vi "build status string.vi"(1 "SpyMessage{}":T1 {"AckBytes [8]" format="%.0x"; "Data [8]" format="%.0x"; "ArbIDOrHeader" format="%.0x"; "DescriptionID" format="%.0x"; "NetworkID" format="%.0x"}, 2 "timestamp":dbl) -> (0 "string out":string)   [LabVIEW 2009]
doc: "this vi builds the string that to be displayed from the received messages.\n\n1/04/2010 1.0.0 jyg\n-initial release"
uses:
  ctl spymessage.ctl
  ctl StatusBitfield.ctl
  ctl spy protocols.ctl
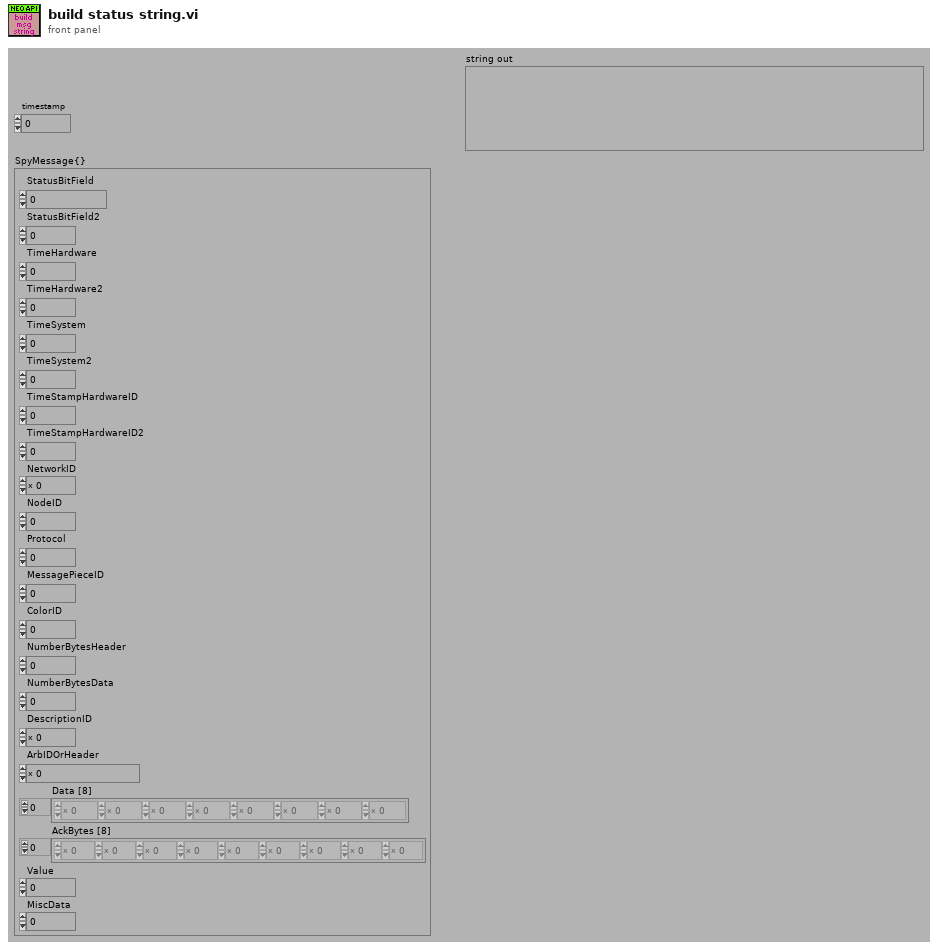
[diagram p1: front panel]
types:
  T1 = typedef "ctl spymessage.ctl" = cluster{"StatusBitField":u32, "StatusBitField2":u32, "TimeHardware":u32, "TimeHardware2":u32, "TimeSystem":u32, "TimeSystem2":u32, "TimeStampHardwareID":u8, "TimeStampHardwareID2":u8, "NetworkID":u8, "NodeID":u8, "Protocol":u8, "MessagePieceID":u8, "ColorID":u8, "NumberBytesHeader":u8, "NumberBytesData":u8, "DescriptionID":u16, "ArbIDOrHeader":u32, "Data [8]":u8[], "AckBytes [8]":u8[], "Value":sgl, "MiscData":u8}
  T2 = typedef "ctl spy protocols.ctl" = enum16{"CUSTOM", "CAN", "GMLAN", "J1850VPW", "J1850PWM", "ISO9141", "Keyword2000", "GM_ALDL_UART", "CHRYSLER_CCD", "CHRYSLER_SCI", "FORD_UBP", "BEAN", "LIN"}
  T3 = typedef "ctl StatusBitfield.ctl" = enum32{"GlobalError", "Tx", "XtdFrame", "RemoteFrame", "ErrCRCError", "CANErrorPassive", "ErrIncompleteFrame", "ErrLostArbitration", "Undefined", "CANBusOff", "CANErrorWarning", "BusShortedPlus", "BusShortedGnd", "CheckSumError", "ErrBadMessageBitTimeError", "IFRData", "HardwareCommError", "ExpectedLengthError", "IncomingNoMatch", "Break", "AVT_VSIRecOverflow", "TestTrigger", "AudioCommentType", "GPSDataValue", "AnalogDigitalInputValue", "TextCommentType", "NetworkMessageType", "VSI_TxUnderRun", "VSI_IFR_CRCBit", "StatusInitMessage", "HighSpeed"}
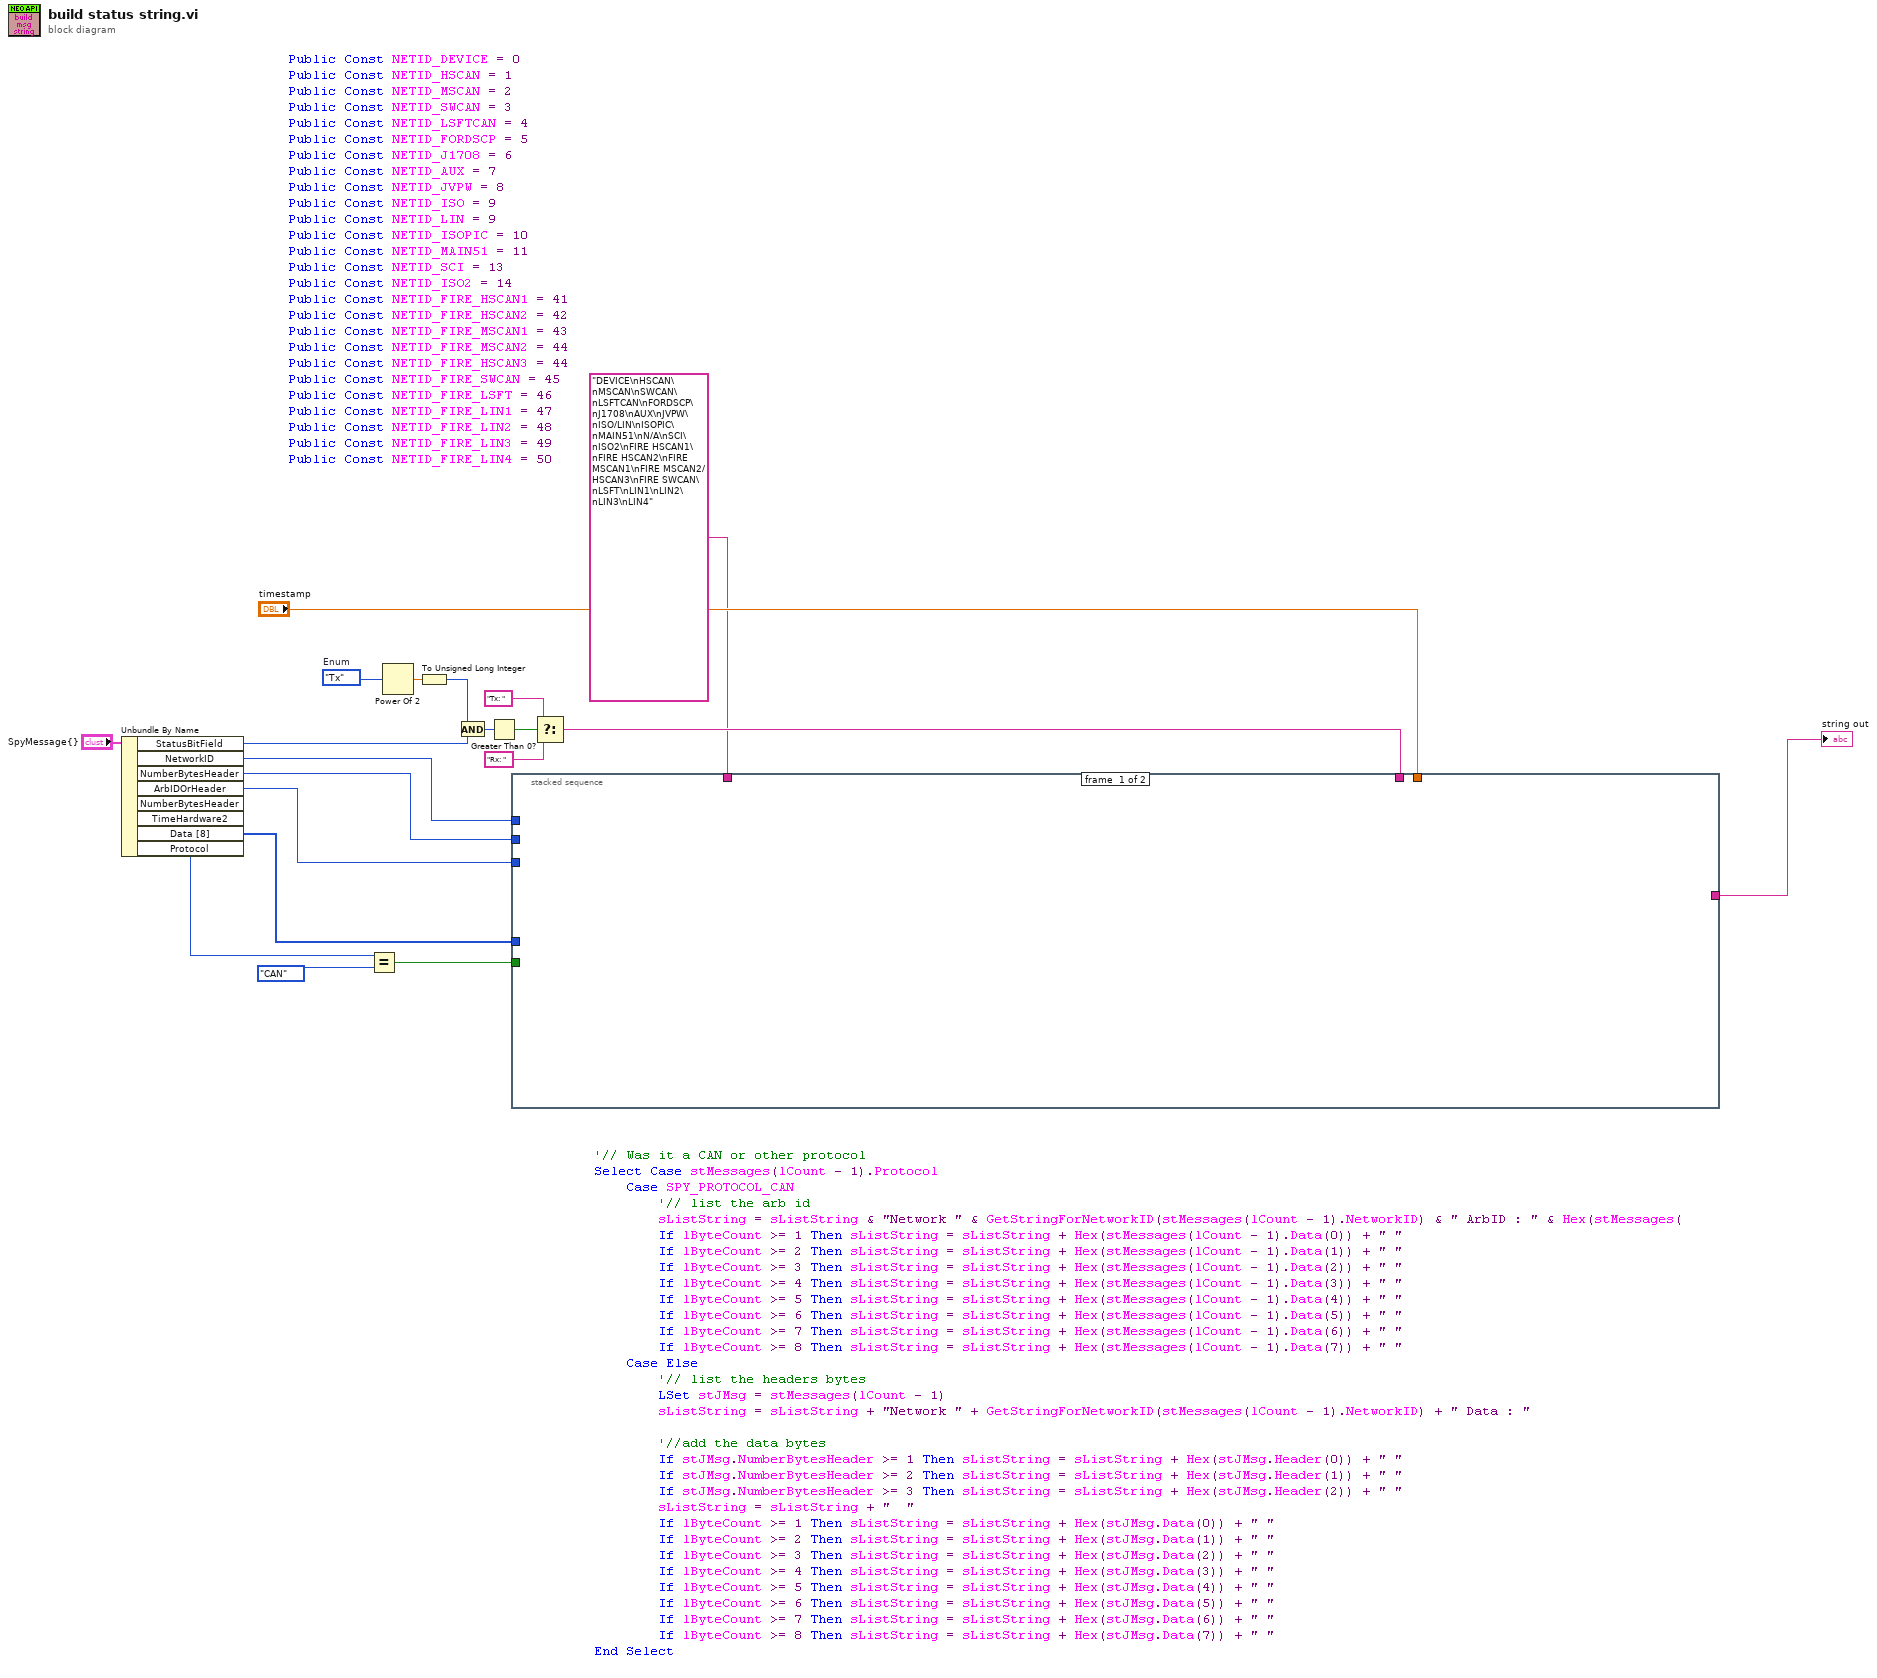
[diagram p0: block diagram]
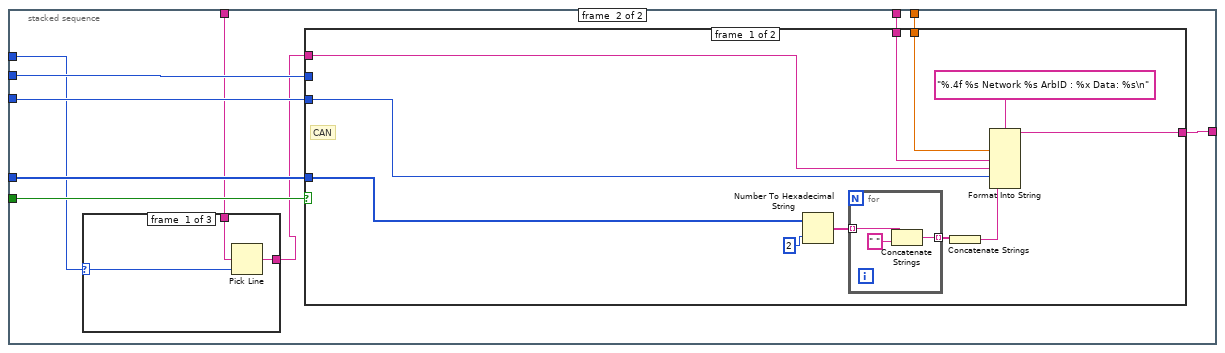
[diagram p2: hidden frame]
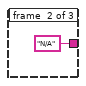
[diagram p3: hidden frame]
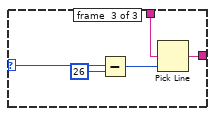
[diagram p4: hidden frame]
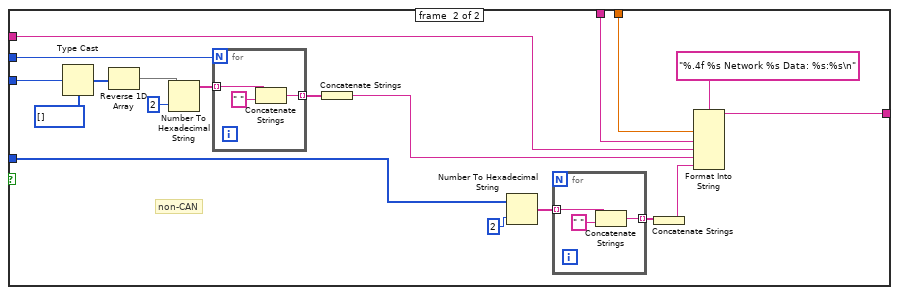
[diagram p5: hidden frame]
diagram:
  w5 = ctl_StatusBitfield."Tx"  # Enum
  n1 = Unbundle By Name("SpyMessage{}") -> ("StatusBitField"=w2:u32, "NetworkID"=w6:u8, "NumberBytesHeader"=w7:u8, "ArbIDOrHeader"=w10:u32, "Data [8]"=w8:u8[], "Protocol"=w15:u8)  [unwired: 2 out]
  n2 = Equal?(x=w15, y=ctl_spy_protocols."CAN" ("Protocol")) -> (x = y?=w13:bool)
  n3 = Power Of 2(x=w5) -> (2^x=w4:dbl)
  n4 = To Unsigned Long Integer(number=w4) -> (unsigned 32bit integer=w3:u32)
  n5 = And(x=w3, y=w2) -> (x .and. y?=w16:u32)
  n6 = Greater Than 0?(x=w16) -> (x > 0?=w17:bool)
  n7 = Select(t="Tx: ", s=w17, f="Rx: ") -> (s? t:f=w11:string)
  n8 = stacked-sequence {
    tunnel: w13 -> [_ w30]
    tunnel: "timestamp" -> [_ w29]
    tunnel: w11 -> [_ w28]
    tunnel: w6 -> [_ w23]
    tunnel: w10 -> [_ w27]
    tunnel: [_ w26] -> w9
    tunnel: w8 -> [_ w25]
    tunnel: w7 -> [_ w24]
    tunnel: "DEVICE\nHSCAN\nMSCAN\nSWCAN\nLSFTCAN\nFORDSCP\nJ1708\nAUX\nJVPW\nISO/LIN\nISOPIC\nMAIN51\nN/A\nSCI\nISO2\nFIRE HSCAN1\nFIRE HSCAN2\nFIRE MSCAN1\nFIRE MSCAN2/HSCAN3\nFIRE SWCAN\nLSFT\nLIN1\nLIN2\nLIN3\nLIN4" -> [_ w22]
    frame #0 {
    }
    frame #1 {
      n9 = case shown="0..14" w23 {
        selector: w23 -> [w32 _ w38]
        tunnel: w22 -> [w33 _ w36]
        tunnel: [w31 "N/A" ("output string") w35] -> w21
        frame #0 {
          n10 = Pick Line(multi-line string=w33, line index=w32) -> (output string=w31:string)  [unwired: 1 out]
        }
        frame #1 {
        }
        frame #2 {
          n11 = Subtract(x=w38, y=u8 26) -> (x-y=w37:u8)
          n12 = Pick Line(multi-line string=w36, line index=w37) -> (output string=w35:string)  [unwired: 1 out]
        }
      }
      n13 = case shown="False" w30 {
        tunnel: w29 -> [w48 w70]
        tunnel: w28 -> [w47 w69]
        tunnel: w27 -> [w46 w65]
        tunnel: [w45 w68] -> w26
        tunnel: w25 -> [w44 w57]
        tunnel: w24 -> [_ w61]
        tunnel: w21 -> [w40 w56]
        frame #0 {
          # "CAN"
          n14 = Number To Hexadecimal String(1:i16 2 ("width (-)"), 2:w44) -> (0:w43:string[])
          n15 = for {
            tunnel: w43 -> [w53] mode=indexing
            tunnel: [w51] -> w42 mode=indexing
            n16 = Concatenate Strings(w53, " " ("string")) -> (w51:string)
          }
          n17 = Concatenate Strings(w42) -> (w41:string)
          n18 = Format Into String(format string="%.4f %s Network %s ArbID : %x Data: %s\n", w48, w47, w40, w46, w41) -> (resulting string=w45:string)  [unwired: 2 in, 1 out]
        }
        frame #1 {
          # "non-CAN"
          n19 = Type Cast(type=u8[] [], x=w65) -> (*(type *) &x=w55:u8[])
          n20 = Reverse 1D Array(array=w55) -> (reversed array=w54:u8[])
          n21 = Number To Hexadecimal String(1:i16 2 ("width (-)"), 2:w54) -> (0:w62:string[])
          n22 = for {
            N: w61 -> [_]
            tunnel: w62 -> [w75] mode=indexing
            tunnel: [w73] -> w60 mode=indexing
            n23 = Concatenate Strings(w75, " " ("string")) -> (w73:string)
          }
          n24 = Concatenate Strings(w60) -> (w59:string)
          n25 = Number To Hexadecimal String(1:i16 2 ("width (-)"), 2:w57) -> (0:w67:string[])
          n26 = for {
            tunnel: w67 -> [w78] mode=indexing
            tunnel: [w76] -> w66 mode=indexing
            n27 = Concatenate Strings(w78, " " ("string")) -> (w76:string)
          }
          n28 = Concatenate Strings(w66) -> (w58:string)
          n29 = Format Into String(format string="%.4f %s Network %s Data: %s:%s\n", w70, w69, w56, w59, w58) -> (resulting string=w68:string)  [unwired: 2 in, 1 out]
        }
      }
    }
  }
  "string out" <- w9
